vi "Laplace Moments.vi"(9 "b":dbl=1.0, 10 "a":dbl=1.0) -> (0 "error":i32, 2 "variance":dbl=2.0, 3 "mean":dbl=1.0)   [LabVIEW 2017, in "NI_Gmath.lvlib"]
doc: "Returns the expected mean and variance of the random variate X, where X describes the selected distribution type. You must manually select the polymorphic instance to use."
uses:
  NI_Gmath.lvlib
  st_error_code.ctl
panel:
  # "Laplace Moments"
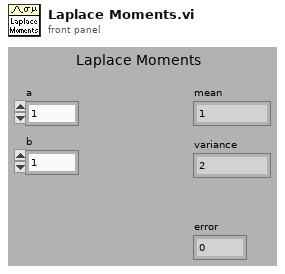
[diagram p1: front panel]
types:
  T1 = typedef "NI_Gmath.lvlib/st_error_code.ctl" = i32
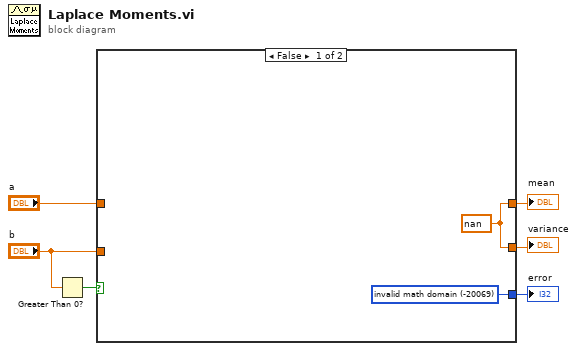
[diagram p0: block diagram]
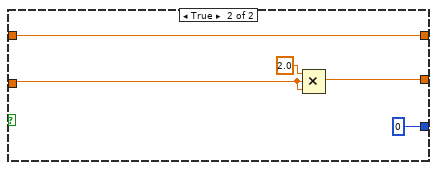
[diagram p2: hidden frame]
diagram:
  n1 = Greater Than 0?(x="b") -> (x > 0?=w2:bool)
  n2 = case shown="False" w2 {
    tunnel: [w7 0 ("invalid math domain")] -> w4
    tunnel: [w8 w12] -> w5
    tunnel: [w8 w11] -> w6
    tunnel: "a" -> [_ w12]
    tunnel: "b" -> [_ w9]
    frame False {
      w7 = T1 -20069 items=["invalid math domain"=-20069, "Fourier interpolation size m >= n"=-20070, "empty array"=-20003] ("stat interp error code")
      w8 = nan
    }
    frame True {
      n3 = Compound Arithmetic op=MULTIPLY(2.0 ("value"), w9, w9) -> (w11:dbl)
    }
  }
  "mean" <- w5
  "error" <- w4
  "variance" <- w6
